vi "ScatTheory.vi"(0 "Tranducer Info":T5={"bandwidth"=4.5, "center freq"=5.75, "start freq"=0.0, "ID"=0} {"bandwidth" format="%.2f"; "center freq" format="%.2f"; "start freq" format="%.2f"}, 1 "Calc type":enum32{"find spec params", "find cq^2"}(tab), 5 "Data System params":T1={"sample freq (MHz)"=50.0, "focal length (mm)"=32.0, "aperature radius (mm)"=3.5, "pts in window"=64.0} {"pts in window" format="%.2f"; "aperature radius (mm)" format="%.2f"; "focal length (mm)" format="%.2f"; "sample freq (MHz)" format="%.2f"}, 7 "material props":T2={"sound speed mm/micros"=1.54, "particle Z"=0.0, "host Zo"=1.0, "scatterer"=0} {"scatterer" items=["isotropic", "cylindrical", "planar"]; "host Zo" format="%.2f"; "particle Z" format="%.2f"; "sound speed mm/micros" format="%.2f"}, 9 "slope":dbl format="%.2f", 11 "midband":dbl format="%.2f", 12 "con (part/cc)":dbl=1.0 format="%.2f", 13 "radius (mm)":dbl format="%.2f") -> (4 "spectral params":T3 {"midband" format="%.2f"; "slope" format="%.2f"; "intercept" format="%.2f"}, 10 "particle size params":T4 {"radius (mm)" format="%.2f"; "cq^2" format="%.2f"; "c (part/cc)" format="%.2f"})   [LabVIEW 2022 SP3]
panel:
  out "gate length (mm)":dbl format="%.2f"
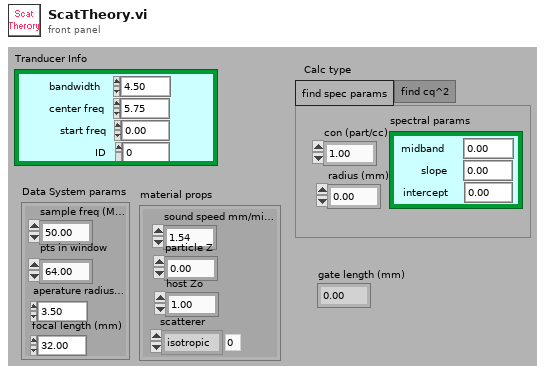
[diagram p1: front panel]
types:
  T1 = cluster{"sample freq (MHz)":dbl, "focal length (mm)":sgl, "aperature radius (mm)":sgl, "pts in window":dbl}
  T2 = cluster{"sound speed mm/micros":dbl, "particle Z":dbl, "host Zo":dbl, "scatterer":i32}
  T3 = cluster{"midband":sgl, "slope":sgl, "intercept":sgl}
  T4 = cluster{"radius (mm)":sgl, "cq^2":ext, "c (part/cc)":ext}
  T5 = cluster{"bandwidth":sgl, "center freq":sgl, "start freq":sgl, "ID":i32}
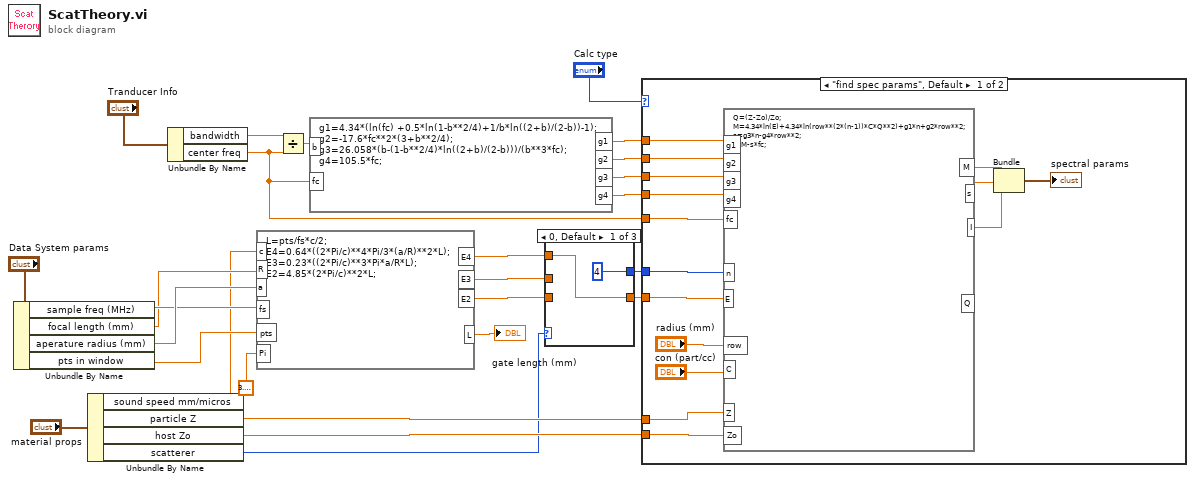
[diagram p0: block diagram]
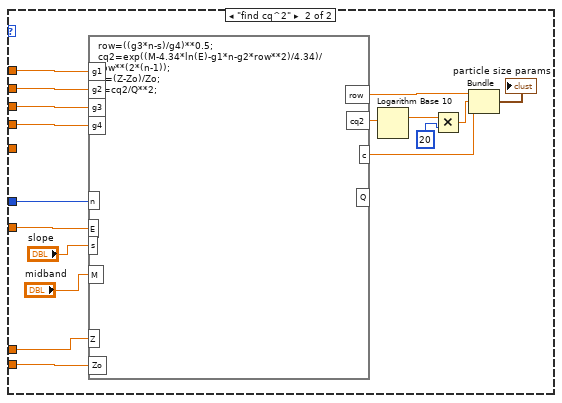
[diagram p2: hidden frame]
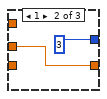
[diagram p3: hidden frame]
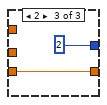
[diagram p4: hidden frame]
diagram:
  n1 = Unbundle By Name("Data System params") -> ("sample freq (MHz)"=w8:dbl, "focal length (mm)"=w7:sgl, "aperature radius (mm)"=w9:sgl, "pts in window"=w10:dbl)
  n2 = Unbundle By Name("material props") -> ("sound speed mm/micros"=w5:dbl, "particle Z"=w4:dbl, "host Zo"=w3:dbl, "scatterer"=w2:i32)
  n3 = Unbundle By Name("Tranducer Info") -> ("bandwidth"=w22:sgl, "center freq"=w14:sgl)
  n4 = formula code="L=pts/fs*c/2;\nE4=0.64*((2*Pi/c)**4*Pi/3*(a/R)**2*L);\nE3=0.23*((2*Pi/c)**3*Pi*a/R*L);\nE2=4.85*(2*Pi/c)**2*L;"("c"=w5, "R"=w7, "a"=w9, "fs"=w8, "pts"=w10, "Pi"=3.141592653589793) -> ("E4"=w26:dbl, "E3"=w25:dbl, "E2"=w24:dbl, "L"=→"gate length (mm)":dbl)
  n5 = Divide(x=w22, y=w14) -> (x/y=w21:sgl)
  n6 = formula code="g1=4.34*(ln(fc) +0.5*ln(1-b**2/4)+1/b*ln((2+b)/(2-b))-1);\ng2=-17.6*fc**2*(3+b**2/4);\ng3=26.058*(b-(1-b**2/4)*ln((2+b)/(2-b)))/(b**3*fc);\ng4=105.5*fc;"("b"=w21, "fc"=w14) -> ("g1"=w20:dbl, "g2"=w19:dbl, "g3"=w18:dbl, "g4"=w17:dbl)
  n7 = case shown="0, Default" w2 {
    tunnel: w26 -> [w28 _ _]
    tunnel: w25 -> [_ w29 _]
    tunnel: w24 -> [_ _ w31]
    tunnel: [w28 w29 w31] -> w15
    tunnel: [4 3 2] -> w16
    frame 0, Default {
    }
    frame 1 {
    }
    frame 2 {
    }
  }
  n8 = case shown="\"find spec params\", Default" "Calc type" {
    tunnel: w20 -> [w47 w64]
    tunnel: w19 -> [w46 w63]
    tunnel: w18 -> [w45 w62]
    tunnel: w17 -> [w44 w61]
    tunnel: w16 -> [w43 w60]
    tunnel: w15 -> [w42 w59]
    tunnel: w14 -> [w41 _]
    tunnel: w4 -> [w34 w53]
    tunnel: w3 -> [w33 w52]
    frame "find spec params", Default {
      n9 = formula code="Q=(Z-Zo)/Zo;\nM=4.34*ln(E)+4.34*ln(row**(2*(n-1))*C*Q**2)+g1*n+g2*row**2;\ns=g3*n-g4*row**2;\nI=M-s*fc;"("g1"=w47, "g2"=w46, "g3"=w45, "g4"=w44, "n"=w43, "E"=w42, "row"="radius (mm)", "fc"=w41, "C"="con (part/cc)", "Z"=w34, "Zo"=w33) -> ("M"=w39:dbl, "s"=w38:dbl, "I"=w37:dbl)  [unwired: 1 out]
      n10 = Bundle("M"=w39, "s"=w38, "I"=w37) -> (→"spectral params":cluster{"M":dbl, "s":dbl, "I":dbl})  [unwired: 1 out]
    }
    frame "find cq^2" {
      n11 = formula code="row=((g3*n-s)/g4)**0.5;\ncq2=exp((M-4.34*ln(E)-g1*n-g2*row**2)/4.34)/row**(2*(n-1));\nQ=(Z-Zo)/Zo;\nc=cq2/Q**2;"("g1"=w64, "g2"=w63, "g3"=w62, "g4"=w61, "n"=w60, "E"=w59, "s"="slope", "M"="midband", "Z"=w53, "Zo"=w52) -> ("row"=w58:dbl, "cq2"=w50:dbl, "c"=w57:dbl)  [unwired: 1 out]
      n12 = Logarithm Base 10(1:w50) -> (0:w49:dbl)
      n13 = Multiply(x=w49, y=20) -> (x*y=w51:dbl)
      n14 = Bundle("row"=w58, w51, "c"=w57) -> (→"particle size params":cluster{"row":dbl, dbl, "c":dbl})  [unwired: 1 out]
    }
  }
